vi "Save Project.vi"(0 "Project reference":refnum<vi>, 5 "MeasurementCore reference":refnum<vi>, 7 "Project path":path, 11 "error in (no error)":errorcluster) -> (15 "error out":errorcluster)   [LabVIEW 2021, in "Multiple Migrator.lvlib"]
uses:
  Multiple Migrator.lvlib
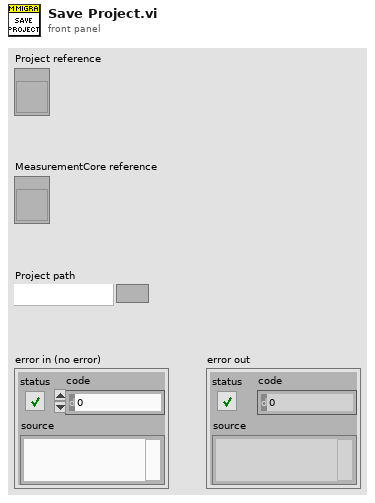
[diagram p1: front panel]
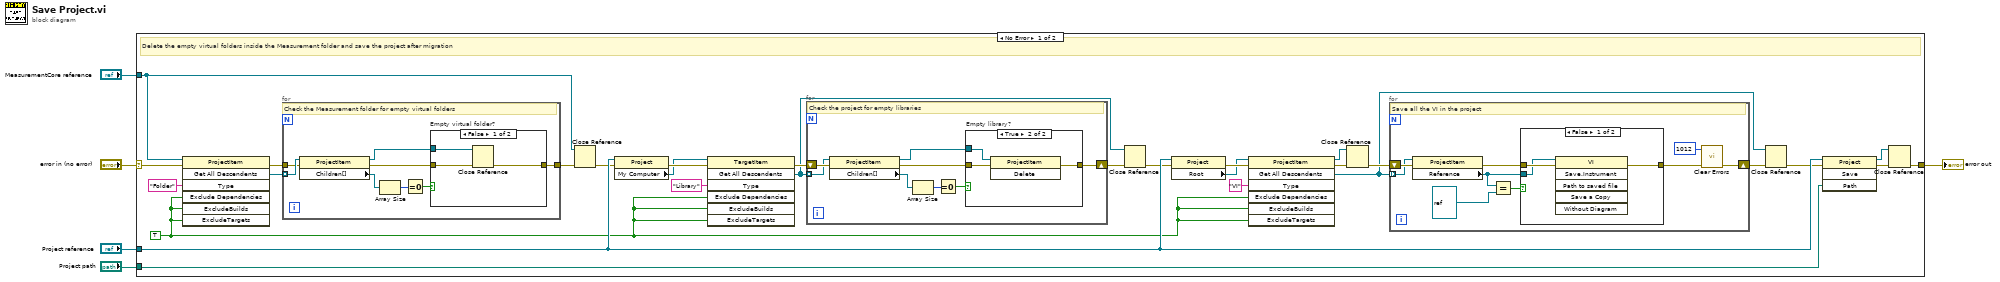
[diagram p0: block diagram]
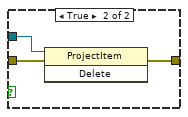
[diagram p2: hidden frame]
diagram:
  n1 = case shown="No Error" "error in (no error)" {
    selector: "error in (no error)" -> [w31 w74]
    tunnel: [w33 w74] -> w5
    tunnel: "Project path" -> [w28 _]
    tunnel: "MeasurementCore reference" -> [w7 _]
    tunnel: "Project reference" -> [w18 _]
    frame No Error {
      w6 = TRUE
      # "Delete the empty virtual folders inside the Measurement folder and save the project after migration"
      n2 = invoke class="ProjectItem" method="Get All Descendents"(reference=w7, error in=w31, "Type"="Folder", "Exclude Dependencies"=w6, "ExcludeBuilds"=w6, "ExcludeTargets"=w6) -> (error out=w29:errorcluster, "All Descendents"=w17:refnum<vi>[])  [unwired: 1 in, 5 out]
      n3 = for {
        tunnel: w17 -> [w42] mode=indexing
        tunnel: w29 -> [w41]
        tunnel: [w35] -> w9
        # "Check the Measurement folder for empty virtual folders"
        n4 = property class="ProjectItem"(reference=w42, error in=w41) -> (reference out=w36:refnum<vi>, error out=w38:errorcluster, "Children[]"=w40:refnum<vi>[])
        n5 = Array Size(array=w40) -> (size(s)=w39:i32)
        n6 = Equal To 0?(x=w39) -> (x = 0?=w37:bool)
        n7 = case "Empty virtual folder?" shown="False" w37 {
          tunnel: w38 -> [w45 w48]
          tunnel: w36 -> [w44 w47]
          tunnel: [w43 w46] -> w35
          frame False {
            n8 = Close Reference(reference=w44, error in (no error)=w45) -> (error out=w43:errorcluster)
          }
          frame True {
            n9 = invoke class="ProjectItem" method="Delete"(reference=w47, error in=w48) -> (error out=w46:errorcluster)  [unwired: 1 in, 2 out]
          }
        }
      }
      n10 = Close Reference(reference=w7, error in (no error)=w9) -> (error out=w8:errorcluster)
      n11 = property class="Project"(reference=w18, error in=w8) -> (error out=w22:errorcluster, "My Computer"=w11:refnum<vi>)  [unwired: 1 out]
      n12 = invoke class="TargetItem" method="Get All Descendents"(reference=w11, error in=w22, "Type"="Library", "Exclude Dependencies"=w6, "ExcludeBuilds"=w6, "ExcludeTargets"=w6) -> (error out=w20:errorcluster, "All Descendents"=w15:refnum<vi>[])  [unwired: 1 in, 5 out]
      n13 = for {
        shift-right: [w49] -> w16
        shift-left: w20 -> [w56]
        tunnel: w15 -> [w55] mode=indexing
        # "Check the project for empty libraries"
        n14 = property class="ProjectItem"(reference=w55, error in=w56) -> (reference out=w51:refnum<vi>, error out=w50:errorcluster, "Children[]"=w53:refnum<vi>[])
        n15 = Array Size(array=w53) -> (size(s)=w54:i32)
        n16 = Equal To 0?(x=w54) -> (x = 0?=w52:bool)
        n17 = case "Empty library?" shown="True" w52 {
          tunnel: w50 -> [w57 w60]
          tunnel: w51 -> [_ w59]
          tunnel: [w57 w58] -> w49
          frame False {
          }
          frame True {
            n18 = invoke class="ProjectItem" method="Delete"(reference=w59, error in=w60) -> (error out=w58:errorcluster)  [unwired: 1 in, 2 out]
          }
        }
      }
      n19 = Close Reference(reference=w15, error in (no error)=w16) -> (error out=w10:errorcluster)
      n20 = property class="Project"(reference=w18, error in=w10) -> (error out=w27:errorcluster, "Root"=w26:refnum<vi>)  [unwired: 1 out]
      n21 = invoke class="ProjectItem" method="Get All Descendents"(reference=w26, error in=w27, "Type"="VI", "Exclude Dependencies"=w6, "ExcludeBuilds"=w6, "ExcludeTargets"=w6) -> (reference out=w24:refnum<vi>, error out=w25:errorcluster, "All Descendents"=w12:refnum<vi>[])  [unwired: 1 in, 4 out]
      n22 = Close Reference(reference=w24, error in (no error)=w25) -> (error out=w23:errorcluster)
      n23 = for {
        shift-right: [w62] -> w14
        shift-left: w23 -> [w68]
        tunnel: w12 -> [w66] mode=indexing
        # "Save all the VI in the project"
        n24 = property class="ProjectItem"(reference=w66, error in=w68) -> (error out=w67:errorcluster, "Reference"=w63:refnum<vi>)  [unwired: 1 out]
        n25 = Equal?(x=w63, y=refnum<vi> refnum) -> (x = y?=w64:bool)
        n26 = case shown="False" w64 {
          tunnel: [w70 w73] -> w69
          tunnel: w67 -> [w72 w73]
          tunnel: w63 -> [w71 _]
          frame False {
            n27 = invoke class="VI" method="Save.Instrument"(reference=w71, error in=w72) -> (error out=w70:errorcluster)  [unwired: 4 in, 5 out]
          }
          frame True {
          }
        }
        n28 = call <vilib>:"Clear Errors.vi"("error in (no error)"=w69, "specific error code to clear (0: all)"=1012) -> ("error out"=w62:errorcluster)  [unwired: 4 in, 1 out]
      }
      n29 = Close Reference(reference=w12, error in (no error)=w14) -> (error out=w13:errorcluster)
      n30 = invoke class="Project" method="Save"(reference=w18, error in=w13, "Path"=w28) -> (reference out=w34:refnum<vi>, error out=w32:errorcluster)  [unwired: 1 in, 2 out]
      n31 = Close Reference(reference=w34, error in (no error)=w32) -> (error out=w33:errorcluster)
    }
    frame Error {
    }
  }
  "error out" <- w5
